vi "commands.vi"() -> ()   [LabVIEW 2018]
panel:
  out "Joystick_Driver-B":bool
  out "Joystick_Driver-A":bool
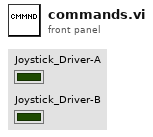
[diagram p1: front panel]
diagram:
